vi "Queue.vi"() -> ()   [LabVIEW 2018]
panel:
  in  "정지 버튼":bool
  in  "큐 팝 속도":u16(ring) items=["100", "500"]
  in  "큐 삽입 속도":u16(ring) items=["100", "500"]
  out "수직 채움 슬라이드":dbl(slide) scale=0.0..50.0
  out "큐 pop":dbl(graph)
  out "큐 삽입":dbl(graph)
  out "웨이브폼 차트 4":dbl(graph)
  in  "정지 3":bool
  out "웨이브폼 차트 3":dbl(graph)
  in  "정지 2":bool
  out "웨이브폼 차트 2":dbl(graph)
  out "웨이브폼 차트":dbl(graph)
  in  "정지":bool
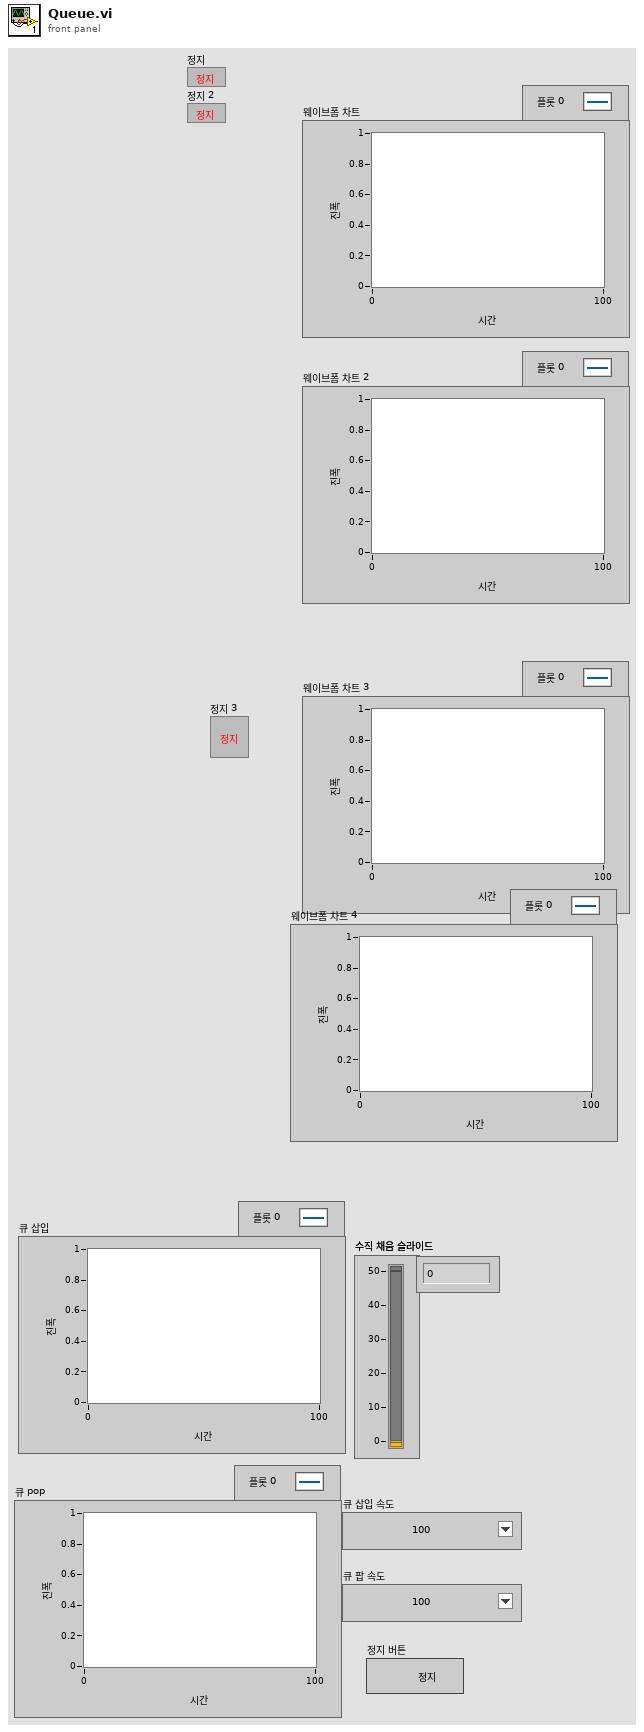
[diagram p1: front panel]
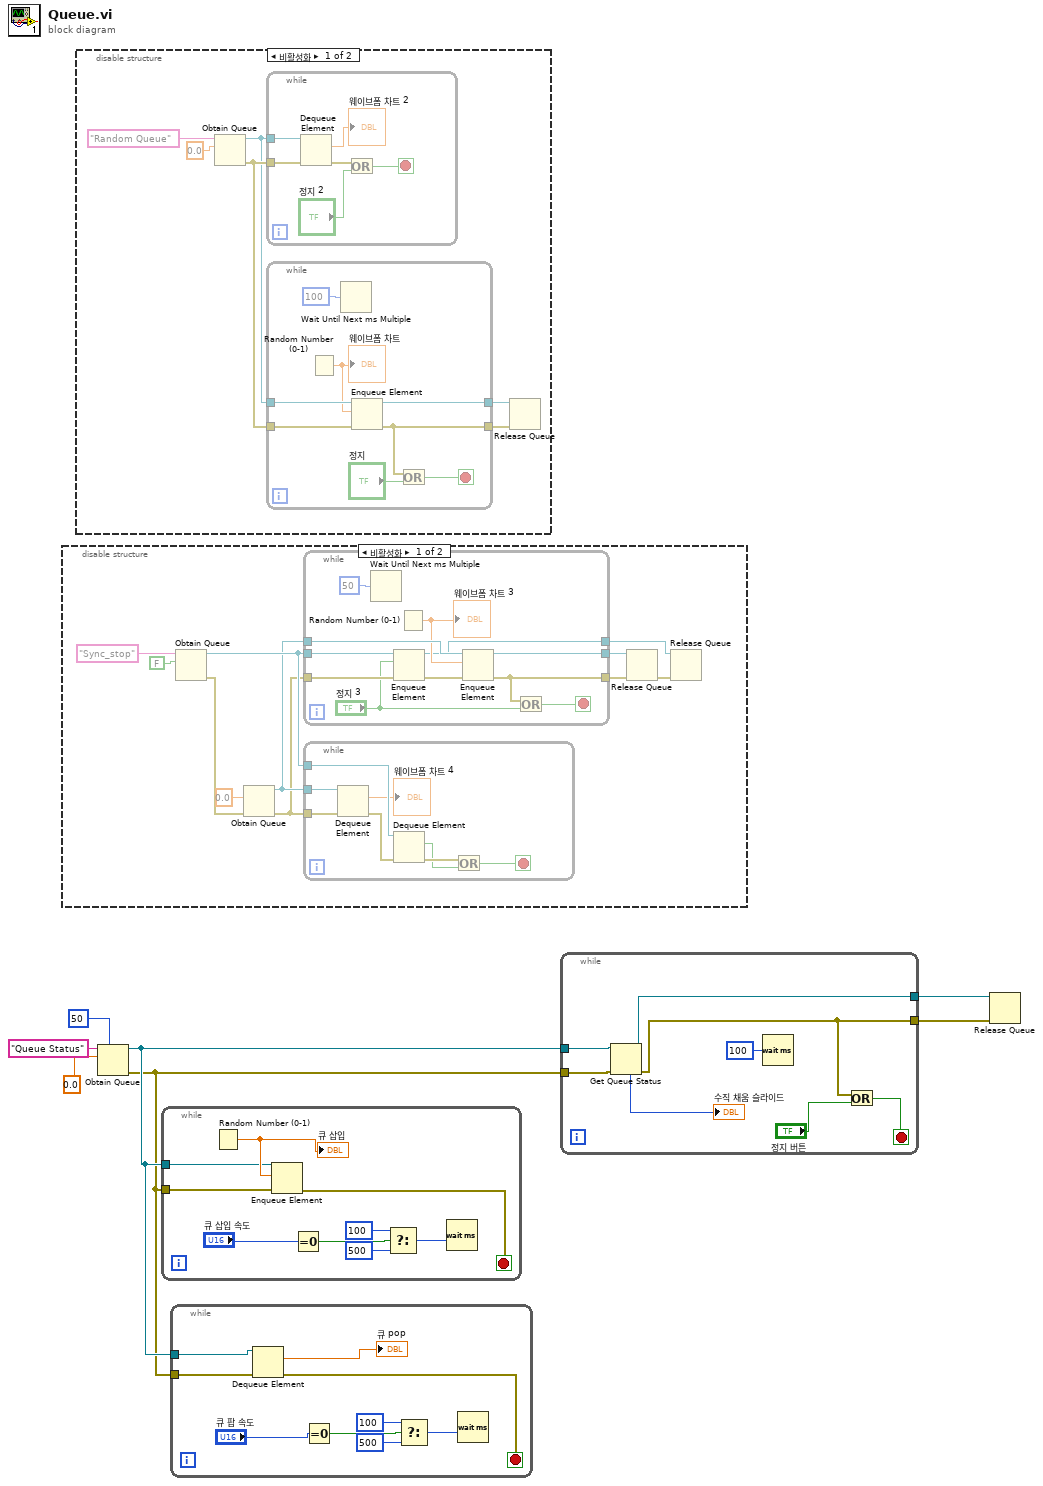
[diagram p0: block diagram]
diagram:
  n1 = disable-structure shown="비활성화" {
    frame Disabled {
      n2 = Obtain Queue(name (unnamed)="Sync_stop" ("이름(이름없음)"), element data type=FALSE) -> (queue out=w11:refnum<queue>, error out=w9:errorcluster)  [unwired: 3 in, 1 out]
      n3 = Obtain Queue(element data type=0.0, error in (no error)=w9) -> (queue out=w10:refnum<queue>, error out=w8:errorcluster)  [unwired: 3 in, 1 out]
      n4 = while {
        tunnel: w11 -> [w37]
        tunnel: w10 -> [w36]
        tunnel: w8 -> [w32]
        tunnel: [w30] -> w15
        tunnel: [w29] -> w14
        tunnel: [w28] -> w12
        stop <- w33 stop-if-true
        n5 = Wait Until Next ms Multiple(millisecond multiple=u32 50 ("ms 배수")) -> ()  [unwired: 1 out]
        n6 = Enqueue Element(queue=w37, element="정지 3", error in (no error)=w32) -> (queue out=w30:refnum<queue>, error out=w31:errorcluster)  [unwired: 1 in, 1 out]
        n7 = Random Number (0-1)() -> (number: 0 to 1=w34:dbl)
        "웨이브폼 차트 3" <- w34
        n8 = Enqueue Element(queue=w36, element=w34, error in (no error)=w31) -> (queue out=w28:refnum<queue>, error out=w29:errorcluster)  [unwired: 1 in, 1 out]
        n9 = Or(x=w29, y="정지 3") -> (x .or. y?=w33:bool)
      }
      n10 = while {
        tunnel: w11 -> [w21]
        tunnel: w10 -> [w22]
        tunnel: w8 -> [w26]
        stop <- w23 stop-if-true
        n11 = Dequeue Element(queue=w22, error in (no error)=w26) -> (element=→"웨이브폼 차트 4":dbl, error out=w25:errorcluster)  [unwired: 1 in, 2 out]
        n12 = Dequeue Element(queue=w21, error in (no error)=w25) -> (element=w20:bool, error out=w24:errorcluster)  [unwired: 1 in, 2 out]
        n13 = Or(x=w24, y=w20) -> (x .or. y?=w23:bool)
      }
      n14 = Release Queue(queue=w12, error in (no error)=w14) -> (error out=w13:errorcluster)  [unwired: 1 in, 2 out]
      n15 = Release Queue(queue=w15, error in (no error)=w13) -> ()  [unwired: 1 in, 3 out]
    }
    frame Enabled {
    }
  }
  n16 = disable-structure shown="비활성화" {
    frame Disabled {
      n17 = Obtain Queue(name (unnamed)="Random Queue" ("이름(이름없음)"), element data type=0.0) -> (queue out=w38:refnum<queue>, error out=w39:errorcluster)  [unwired: 3 in, 1 out]
      n18 = while {
        tunnel: w38 -> [w49]
        tunnel: w39 -> [w47]
        stop <- w44 stop-if-true
        n19 = Dequeue Element(queue=w49, error in (no error)=w47) -> (element=→"웨이브폼 차트 2":dbl, error out=w46:errorcluster)  [unwired: 1 in, 2 out]
        n20 = Or(x=w46, y="정지 2") -> (x .or. y?=w44:bool)
      }
      n21 = while {
        tunnel: w38 -> [w57]
        tunnel: [w56] -> w41
        tunnel: w39 -> [w55]
        tunnel: [w54] -> w40
        stop <- w52 stop-if-true
        n22 = Random Number (0-1)() -> (number: 0 to 1=w50:dbl)
        "웨이브폼 차트" <- w50
        n23 = Wait Until Next ms Multiple(millisecond multiple=u32 100 ("ms 배수")) -> ()  [unwired: 1 out]
        n24 = Enqueue Element(queue=w57, element=w50, error in (no error)=w55) -> (queue out=w56:refnum<queue>, error out=w54:errorcluster)  [unwired: 1 in, 1 out]
        n25 = Or(x=w54, y="정지") -> (x .or. y?=w52:bool)
      }
      n26 = Release Queue(queue=w41, error in (no error)=w40) -> ()  [unwired: 1 in, 3 out]
    }
    frame Enabled {
    }
  }
  n27 = Obtain Queue(max queue size (-1, unlimited)=50 ("최대 큐 크기(-1,제한없음)"), name (unnamed)="Queue Status" ("이름(이름없음)"), element data type=0.0) -> (queue out=w4:refnum<queue>, error out=w3:errorcluster)  [unwired: 2 in, 1 out]
  n28 = while {
    tunnel: w4 -> [w65]
    tunnel: w3 -> [w64]
    stop <- w63 stop-if-true
    n29 = Random Number (0-1)() -> (number: 0 to 1=w66:dbl)
    "큐 삽입" <- w66
    n30 = Enqueue Element(queue=w65, element=w66, error in (no error)=w64) -> (error out=w63:errorcluster)  [unwired: 1 in, 2 out]
    n31 = Equal To 0?(x="큐 삽입 속도") -> (x = 0?=w59:bool)
    n32 = Select(t=u16 100, s=w59, f=u16 500) -> (s? t:f=w58:u16)
    n33 = Wait (ms)(milliseconds to wait=w58) -> ()  [unwired: 1 out]
  }
  n34 = while {
    tunnel: w4 -> [w70]
    tunnel: w3 -> [w69]
    stop <- w67 stop-if-true
    n35 = Dequeue Element(queue=w70, error in (no error)=w69) -> (element=→"큐 pop":dbl, error out=w67:errorcluster)  [unwired: 1 in, 2 out]
    n36 = Equal To 0?(x="큐 팝 속도") -> (x = 0?=w74:bool)
    n37 = Select(t=u16 100, s=w74, f=u16 500) -> (s? t:f=w75:u16)
    n38 = Wait (ms)(milliseconds to wait=w75) -> ()  [unwired: 1 out]
  }
  n39 = while {
    tunnel: w4 -> [w83]
    tunnel: w3 -> [w82]
    tunnel: [w79] -> w2
    tunnel: [w80] -> w1
    stop <- w77 stop-if-true
    n40 = Get Queue Status(queue=w83, error in (no error)=w82) -> (queue out=w80:refnum<queue>, error out=w79:errorcluster, # elements in queue=→"수직 채움 슬라이드":i32)  [unwired: 1 in, 5 out]
    n41 = Wait (ms)(milliseconds to wait=u32 100 ("대기 시간 (ms)")) -> ()  [unwired: 1 out]
    n42 = Or(x=w79, y="정지 버튼") -> (x .or. y?=w77:bool)
  }
  n43 = Release Queue(queue=w1, error in (no error)=w2) -> ()  [unwired: 1 in, 3 out]
